vi "stepper driver -- wrapper.vi"(4 "motor selector":T1=enum."--", 6 "Instrument Address":refnum<visa-resource-name>="ASRL2::INSTR", 7 "stepper driver action":T3, 10 "speed IN":dbl, 11 "number IN":dbl format="%#_13g") -> (1 "stepper motor state OUT":T2, 2 "speed OUT":dbl, 3 "number OUT":dbl)   [LabVIEW 2018]
uses:
  stepper driver action.ctl
  stepper motor state.ctl
  motor type.ctl
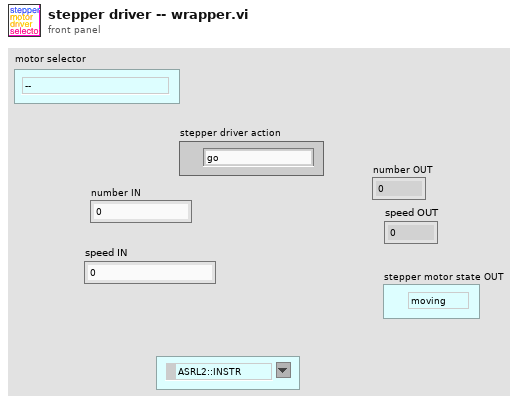
[diagram p1: front panel]
types:
  T1 = typedef "motor type.ctl" = enum16{"IMS", "arduino C&A", "BLM", "--"}
  T2 = typedef "stepper motor state.ctl" = enum16{"moving", "stopped"}
  T3 = typedef "stepper driver action.ctl" = enum16{"go", "void", "stop", "check", "init", "sync", "set", "set speed", "--check status", "--check value", "--handshake"}
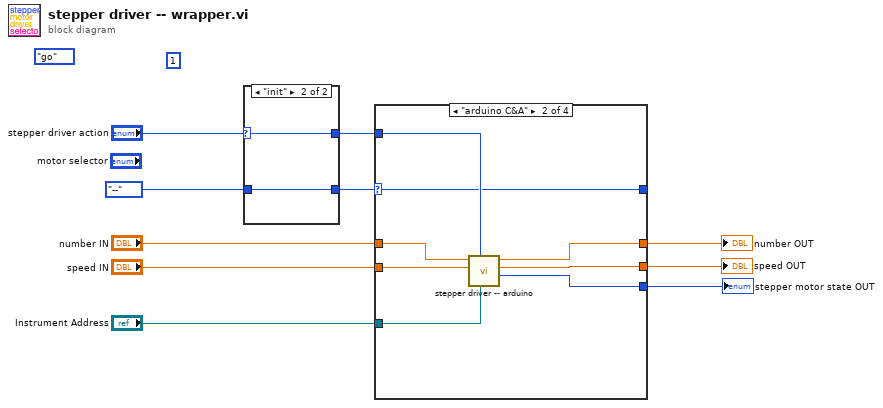
[diagram p0: block diagram]
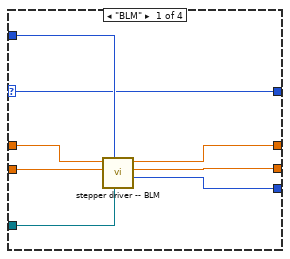
[diagram p3: hidden frame]
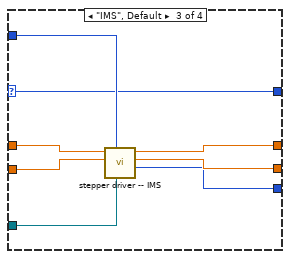
[diagram p4: hidden frame]
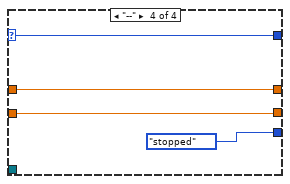
[diagram p5: hidden frame]
diagram:
  (unwired) stepper_driver_action."go" ("stepper driver action")
  (unwired) 1
  n1 = case shown="\"init\"" "stepper driver action" {
    selector: "stepper driver action" -> [w12 w14]
    tunnel: [w12 w14] -> w3
    tunnel: [w11 w13] -> w2
    tunnel: motor_type."--" ("motor selector") -> [w11 w13]
    frame "go", Default {
    }
    frame "init" {
    }
  }
  n2 = case shown="\"arduino C&A\"" w2 {
    selector: w2 -> [w15 w23 w31 w39]
    tunnel: w3 -> [w22 w30 w38 _]
    tunnel: [w21 w29 w37 w41] -> w9
    tunnel: [w20 w28 w36 stepper_motor_state."stopped" ("stepper motor state OUT")] -> w8
    tunnel: [w19 w27 w35 w42] -> w7
    tunnel: "number IN" -> [w18 w26 w34 w42]
    tunnel: "speed IN" -> [w17 w25 w33 w41]
    tunnel: "Instrument Address" -> [w16 w24 w32 _]
    tunnel: [w15 w23 w31 w39] -> _
    frame "BLM" {
      n3 = call "stepper driver -- BLM.vi"("Instrument Address"=w16, "stepper driver action"=w22, "speed IN"=w17, "number"=w18) -> ("stepper motor state OUT"=w20:T2, "speed"=w21:dbl, "number out"=w19:dbl)  [unwired: 5 in]
    }
    frame "arduino C&A" {
      n4 = call "stepper driver -- arduino.vi"("Instrument Address"=w24, "stepper driver action"=w30, "speed IN"=w25, "number"=w26) -> ("stepper motor state OUT"=w28:T2, "speed"=w29:dbl, "number out"=w27:dbl)  [unwired: 5 in]
    }
    frame "IMS", Default {
      n5 = call "stepper driver -- IMS.vi"("Instrument Address"=w32, "stepper driver action"=w38, "speed IN"=w33, "number"=w34) -> ("stepper motor state OUT"=w36:T2, "speed"=w37:dbl, "number out"=w35:dbl)  [unwired: 5 in]
    }
    frame "--" {
    }
  }
  "speed OUT" <- w9
  "stepper motor state OUT" <- w8
  "number OUT" <- w7
